vi "Read configuration.vi"(8 "error in":errorcluster, 11 "CentralErrorHandlerDev editor node in":refnum<class "CentralErrorHandler editor node.lvclass">) -> (0 "error out":errorcluster, 2 "configuration":refnum<class "NISE_CEF_serializable configuration.lvclass">, 3 "CentralErrorHandlerDev editor node out":refnum<class "CentralErrorHandler editor node.lvclass">)   [LabVIEW 2017, in "CentralErrorHandler editor node.lvclass"]
uses:
  CentralErrorHandler editor node.lvclass
  <vilib>/NI/Configuration Framework/serializable configuration/NISE_CEF_serializable configuration.lvclass
  CentralErrorHandler editor node.lvclass/CentralErrorHandler editor node.ctl
  module/configuration/CentralErrorHandler configuration.lvclass
  C:/Program Files (x86)/National Instruments/LabVIEW 2017/vi.lib/NI/Configuration Framework/serializable configuration/NISE_CEF_serializable configuration.lvclass
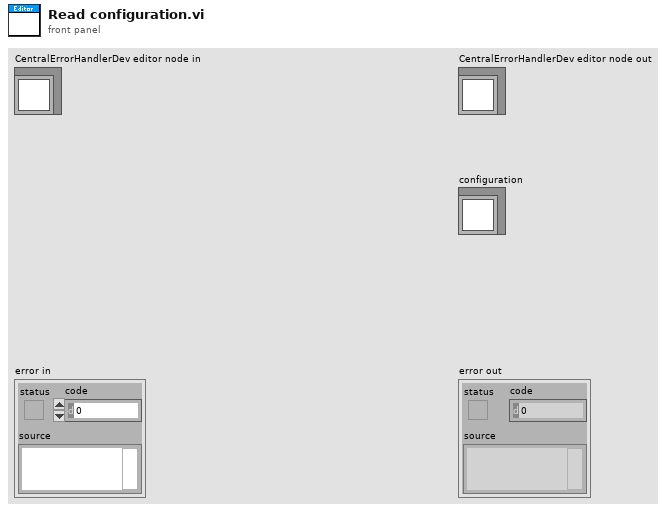
[diagram p1: front panel]
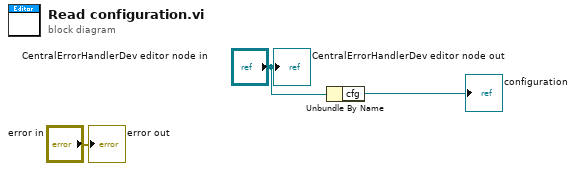
[diagram p0: block diagram]
diagram:
  n1 = Unbundle By Name("CentralErrorHandlerDev editor node in") -> ("cfg"=→"configuration":refnum<class "CentralErrorHandler configuration.lvclass">)
  "error out" <- "error in"
  "CentralErrorHandlerDev editor node out" <- "CentralErrorHandlerDev editor node in"
